vi "TCP IP Connection Timing Tester.vi"() -> ()   [LabVIEW 2015]
panel:
  out "Array":T1(array[cluster])
  out "output cluster":T2
  out "Fornax Connection out":refnum<k5>
  out "error out":errorcluster
  in  "error in (no error)":errorcluster
  in  "Fornax Executable Path":path=path "C:/Program Files (x86)/Medtronic/Fornax/x86/Fornax.exe"
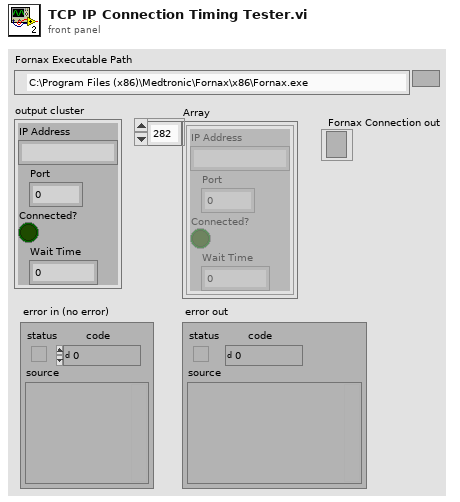
[diagram p1: front panel]
types:
  T1 = cluster{"IP Address":string, "Port":u16, "Connected?":bool, "Wait Time":dbl}[]
  T2 = cluster{"IP Address":string, "Port":u16, "Connected?":bool, "Wait Time":dbl}
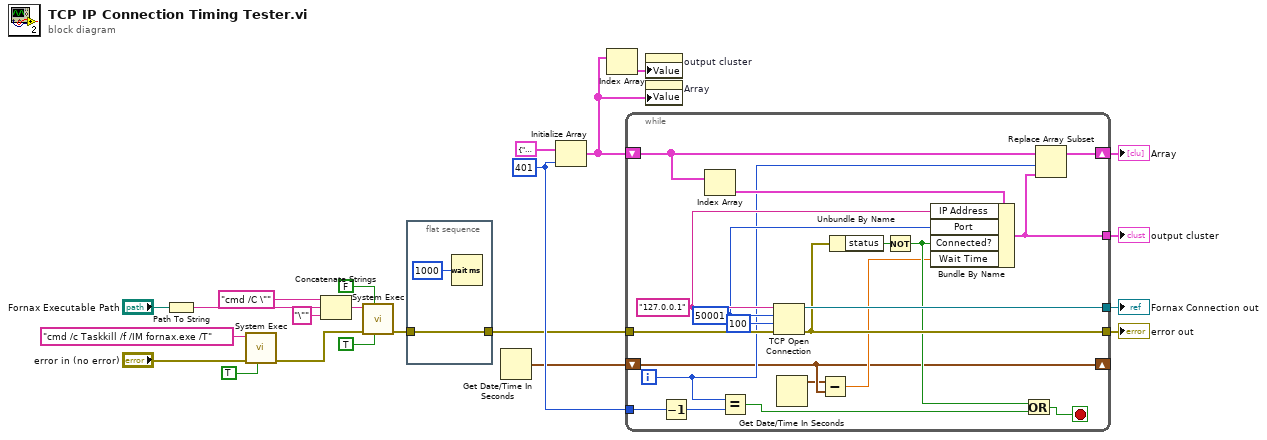
[diagram p0: block diagram]
diagram:
  w18 = 401 ("dimension size")
  n1 = Path To String(path="Fornax Executable Path") -> (string=w7:string)
  n2 = call <vilib>:"System Exec.vi"("run minimized? (F)"=TRUE, "error in (no error)"="error in (no error)", "command line"="cmd /c Taskkill /f /IM fornax.exe /T") -> ("error out"=w13:errorcluster)  [unwired: 5 in, 3 out]
  n3 = Concatenate Strings("cmd /C \"" ("string"), w7, "\"" ("string")) -> (w9:string)
  n4 = call <vilib>:"System Exec.vi"("run minimized? (F)"=TRUE, "wait until completion? (T)"=FALSE, "error in (no error)"=w13, "command line"=w9) -> ("error out"=w1:errorcluster)  [unwired: 4 in, 3 out]
  n5 = flat-sequence {
    tunnel: [w24] -> w2
    tunnel: w1 -> [w24]
    frame #0 {
      n6 = Wait (ms)(milliseconds to wait=u32 1000) -> ()  [unwired: 1 out]
    }
  }
  n7 = Get Date/Time In Seconds() -> (seconds since 1Jan1904=w15:timestamp)
  n8 = Initialize Array(T2 {"IP Address"="", "Port"=0, "Connected?"=FALSE, "Wait Time"=0.0} ("Cluster"), w18) -> (w3:T1)
  n9 = Index Array(array=w3) -> (element=w4:T2)  [unwired: 1 in]
  n10 = while {
    tunnel: [w43] -> w21
    shift-right: [w42] -> w16
    shift-left: w3 -> [w41]
    tunnel: w18 -> [w32]
    tunnel: [w29] -> w17
    shift-right: [w26] -> _
    shift-left: w15 -> [w26]
    tunnel: w2 -> [w44]
    tunnel: [w37] -> w22
    i -> [w28]
    stop <- w34 stop-if-true
    w38 = u16 50001 ("remote port or service name")
    w39 = "127.0.0.1" ("address")
    n11 = Decrement(x=w32) -> (x-1=w31:i32)
    n12 = Index Array(array=w41) -> (element=w40:T2)  [unwired: 1 in]
    n13 = Equal?(x=w28, y=w31) -> (x = y?=w30:bool)
    n14 = TCP Open Connection(address=w39, remote port or service name=w38, timeout ms (60000)=100, error in (no error)=w44) -> (connection ID=w43:refnum<k5>, error out=w37:errorcluster)  [unwired: 1 in]
    n15 = Get Date/Time In Seconds() -> (seconds since 1Jan1904=w25:timestamp)
    n16 = Subtract(x=w25, y=w26) -> (x-y=w27:dbl)
    n17 = Unbundle By Name(w37) -> ("status"=w36:bool)
    n18 = Not(x=w36) -> (.not. x?=w33:bool)
    n19 = Bundle By Name(cluster=w40, "IP Address"=w39, "Port"=w38, "Connected?"=w33, "Wait Time"=w27) -> (w29:T2)
    n20 = Or(x=w33, y=w30) -> (x .or. y?=w34:bool)
    n21 = Replace Array Subset(array=w41, new element=w29, index=w28) -> (w42:T1)
  }
  "error out" <- w22
  "Fornax Connection out" <- w21
  "output cluster" <- w17
  "Array" <- w16
  n22 = property on="output cluster" class="Clust (strict)"("Value"=w4) -> ()  [unwired: 2 in, 2 out]
  n23 = property on="Array" class="Arr (strict)"("Value"=w3) -> ()  [unwired: 2 in, 2 out]
